vi "Get Monitor Queue Status Section and Channels.vi"(8 "error in":errorcluster, 11 "Custom Device Ref in":T1 format="%.0x") -> (0 "error out":errorcluster, 1 "Monitor Queue Status channel Refs":T1[](array[typedef]) format="%.0x", 2 "Monitor Queue Status Section Ref out":T1 format="%.0x", 3 "Custom Device Ref out":T1 format="%.0x", 4 "Found?":bool)   [LabVIEW 2020, in "afdx_custom_device Scripting.lvlib"]
uses:
  afdx_custom_device Scripting.lvlib
  <vilib>/NI VeriStand/Custom Device API/Custom Device Item Ref.ctl
  Constants.vi
  <vilib>/NI VeriStand/Custom Device Tools/Custom Device Utility Library/NI VeriStand - Search for Item by GUID.vi
  <vilib>/NI VeriStand/Custom Device Tools/Custom Device Utility Library/NI VeriStand - Search for Item by Name.vi
  <vilib>/NI VeriStand/Custom Device Tools/Custom Device Utility Library/Custom Device Utility Library.lvlib
  GUID Utility/afdx_custom_device GUID Utility.lvlib
  <vilib>/NI VeriStand/Custom Device API/Custom Device API.lvlib
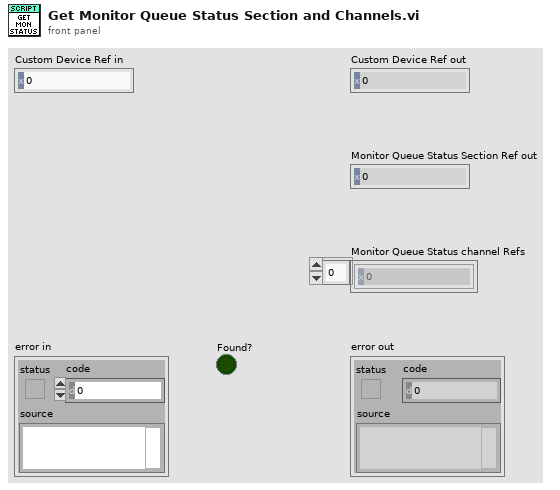
[diagram p1: front panel]
types:
  T1 = typedef "Custom Device API.lvlib/Custom Device Item Ref.ctl" = u64
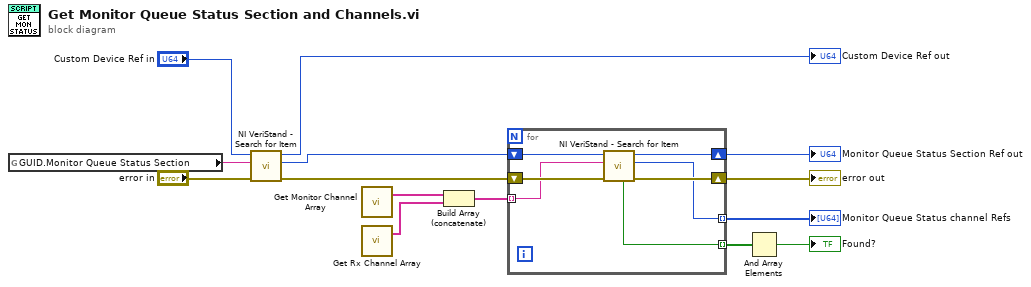
[diagram p0: block diagram]
diagram:
  n1 = global read "Constants.vi" "GUID.Monitor Queue Status Section"() -> (w11:string)
  n2 = call-poly <vilib>:"NI VeriStand - Search for Item.vi"("error in"="error in", "Item GUID"=w11, "Section Ref in"="Custom Device Ref in") -> ("error out"=w12:errorcluster, "Item Ref"=w9:T1, "Section Ref out"=→"Custom Device Ref out":T1)  [unwired: 5 in, 1 out]
  n3 = call "Get Monitor Channel Array.vi"() -> ("Channel Array"=w3:string[])  [unwired: 3 in]
  n4 = call "Get Rx Channel Array.vi"() -> ("Channel Array"=w1:string[])  [unwired: 3 in]
  n5 = Build Array (concatenate)(w3, w1) -> (w2:string[])
  n6 = for {
    tunnel: [w17] -> w6 mode=indexing
    shift-right: [w18] -> w7
    shift-left: w12 -> [w21]
    tunnel: w2 -> [w16] mode=indexing
    shift-right: [w20] -> w10
    shift-left: w9 -> [w19]
    tunnel: [w15] -> w5 mode=indexing
    n7 = call-poly <vilib>:"NI VeriStand - Search for Item.vi"("error in"=w21, "Item Name"=w16, "Section Ref in"=w19) -> ("error out"=w18:errorcluster, "Item Ref"=w17:T1, "Section Ref out"=w20:T1, "Found"=w15:bool)  [unwired: 5 in]
  }
  "Monitor Queue Status Section Ref out" <- w10
  "error out" <- w7
  "Monitor Queue Status channel Refs" <- w6
  n8 = And Array Elements(Boolean array=w5) -> (logical AND=→"Found?":bool)
